vi "SSL_Disconnect.vi"(8 "error in (no error)":errorcluster, 11 "SSL_Connection":T1) -> (0 "error out":errorcluster)   [LabVIEW 2015, in "AWS_IoT.lvlib"]
uses:
  AWS_IoT.lvlib
  Controls/SSL_Connection.ctl
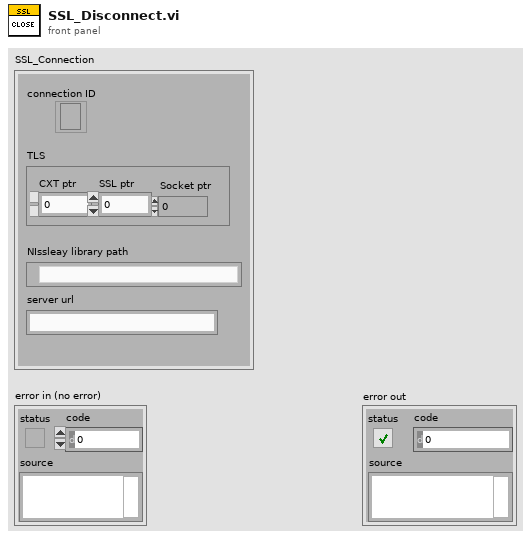
[diagram p1: front panel]
types:
  T1 = typedef "AWS_IoT.lvlib/SSL_Connection.ctl" = cluster{"connection ID":refnum<k5>, "TLS":cluster{"CXT ptr":i32, "SSL ptr":i32, "Socket ptr":u64}, "NIssleay library path":path, "server url":string}
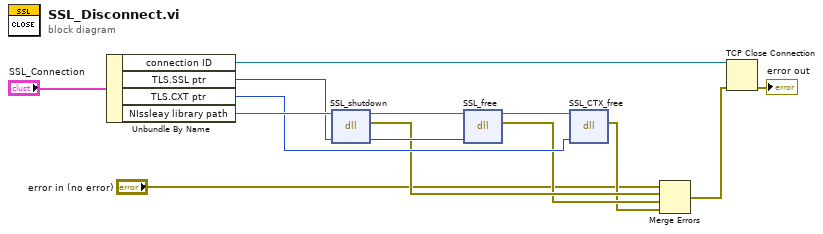
[diagram p0: block diagram]
diagram:
  n1 = Unbundle By Name("SSL_Connection") -> ("connection ID"=w3:refnum<k5>, "TLS.SSL ptr"=w9:i32, "TLS.CXT ptr"=w8:i32, "NIssleay library path"=w11:path)
  n2 = dll-call lib="NIssleay32.*" fn="SSL_shutdown"(path in=w11, "SSL"=w9) -> (path out=w12:path, error out=w7:errorcluster, "SSL"=w10:i32)  [unwired: 3 in]
  n3 = dll-call lib="NIssleay32.*" fn="SSL_free"(path in=w12, "SSL"=w10) -> (path out=w13:path, error out=w6:errorcluster)  [unwired: 4 in]
  n4 = dll-call lib="NIssleay32.*" fn="SSL_CTX_free"(path in=w13, "Context"=w8) -> (error out=w5:errorcluster)  [unwired: 4 in, 1 out]
  n5 = Merge Errors("error in (no error)", w7, w6, w5) -> (w2:errorcluster)
  n6 = TCP Close Connection(connection ID=w3, error in (no error)=w2) -> (error out=→"error out":errorcluster)  [unwired: 1 in, 1 out]
